vi "Check&RPN.vi"(8 "error in (no error)":errorcluster, 11 "Array STEP":T1[](array[typedef])) -> (0 "error out":errorcluster, 3 "Array STEP Out":T1[](array[typedef]))   [LabVIEW 2014, in "SeqLoop.lvlib"]
uses:
  SeqLoop.lvlib
  TypeDefs/STEP.ctl
  TypeDefs/LogicParsedExpression.ctl
  Mimico Display/TypeDefs/Mimic Data.ctl
  Mimico Display/TypeDefs/BG Image.ctl
  Mimico Display/TypeDefs/mObject.ctl
  Mimico Display/Mimico Display.lvlib
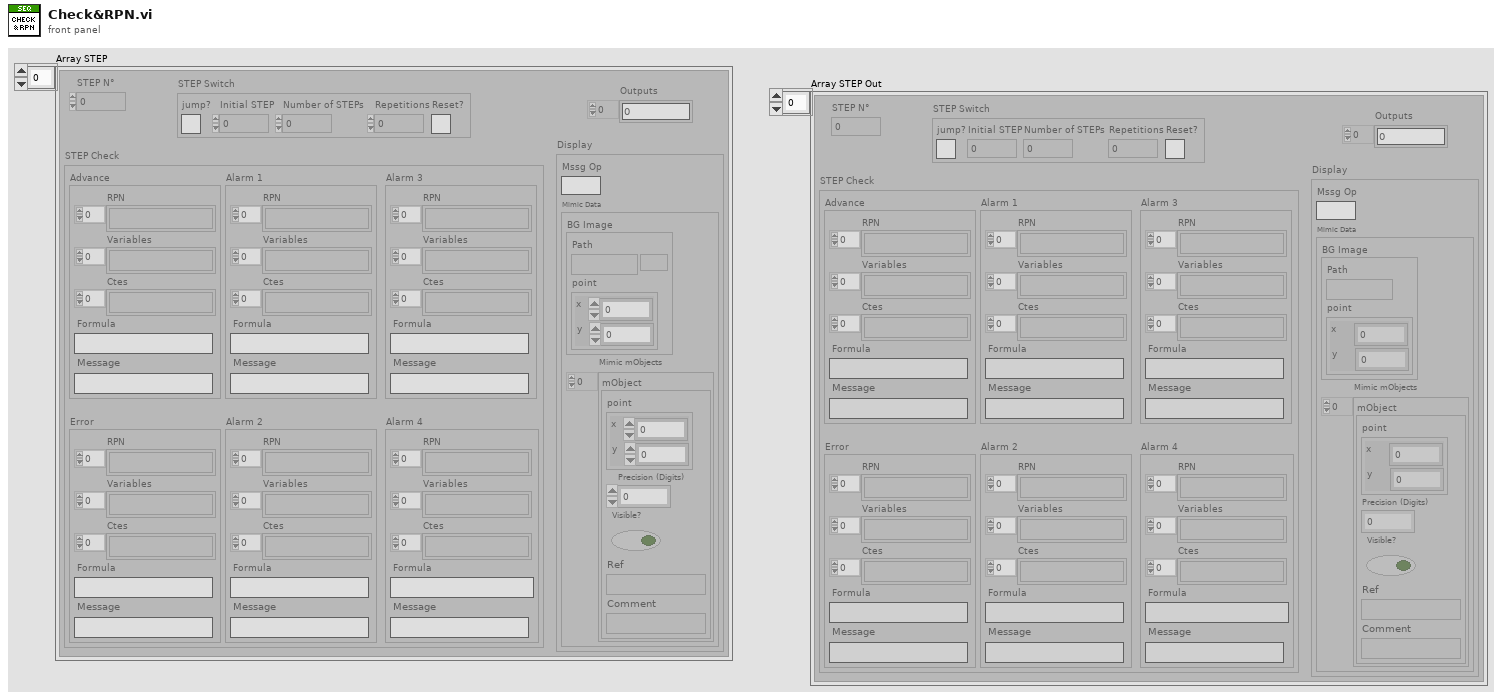
[diagram p1: front panel]
types:
  T1 = typedef "SeqLoop.lvlib/STEP.ctl" = cluster{"STEP N°":u32, "STEP Switch":cluster{"jump?":bool, "Initial STEP":u32, "Number of STEPs":u32, "Repetitions":u32, "Reset?":bool}, "Outputs":i32[], "STEP Check":cluster{"Advance":T2, "Error ":T2, "Alarm 1":T2, "Alarm 2":T2, "Alarm 3":T2, "Alarm 4":T2}, "Display":cluster{"Mssg Op":string, "Mimic Data":T3}}
  T2 = typedef "SeqLoop.lvlib/LogicParsedExpression.ctl" = cluster{"RPN ":string[], "Variables":string[], "Ctes":string[], "Formula":string, "Message":string}
  T3 = typedef "SeqLoop.lvlib/Mimico Display.lvlib/Mimic Data.ctl" = cluster{"BG Image":T4, "Mimic mObjects":T5[]}
  T4 = typedef "SeqLoop.lvlib/Mimico Display.lvlib/BG Image.ctl" = cluster{"Path":path, "point":cluster{"x":i16, "y":i16}}
  T5 = typedef "SeqLoop.lvlib/Mimico Display.lvlib/mObject.ctl" = cluster{"point":cluster{"x":i16, "y":i16}, "Precision (Digits)":i32, "Visible?":bool, "Ref":string, "Comment":string}
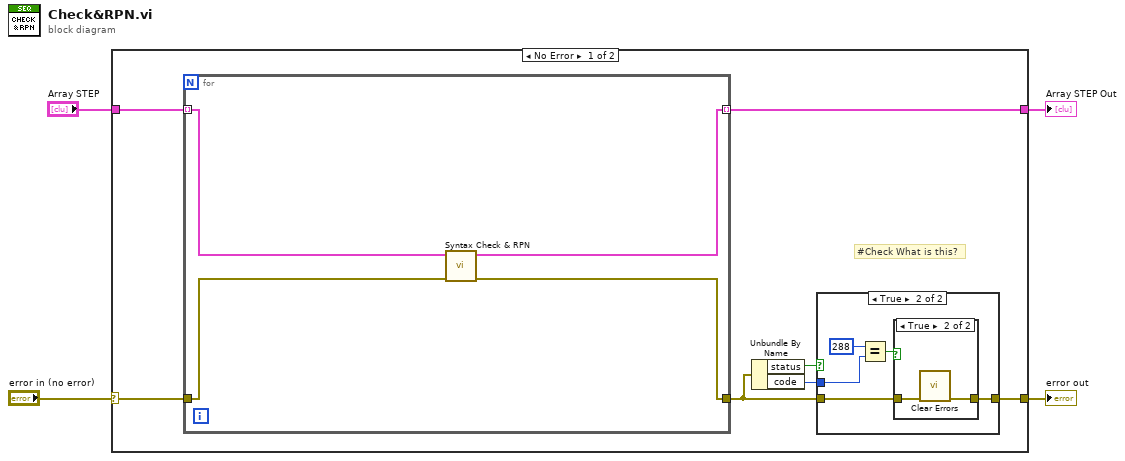
[diagram p0: block diagram]
diagram:
  n1 = case shown="No Error" "error in (no error)" {
    selector: "error in (no error)" -> [w5 w26]
    tunnel: [w8 w26] -> w3
    tunnel: "Array STEP" -> [w6 w25]
    tunnel: [w11 w25] -> w1
    frame No Error {
      # "#Check What is this?"
      n2 = for {
        tunnel: w5 -> [w24]
        tunnel: [w23] -> w7
        tunnel: w6 -> [w22] mode=indexing
        tunnel: [w21] -> w11 mode=indexing
        n3 = call "Syntax Check & RPN.vi"("error in (no error)"=w24, "STEP in"=w22) -> ("error out"=w23:errorcluster, "STEP out"=w21:T1)  [unwired: 8 in]
      }
      n4 = Unbundle By Name(w7) -> ("status"=w9:bool, "code"=w10:i32)
      n5 = case shown="True" w9 {
        tunnel: [w12 w13] -> w8
        tunnel: w7 -> [w12 w14]
        tunnel: w10 -> [_ w17]
        frame False {
        }
        frame True {
          n6 = Equal?(x=288, y=w17) -> (x = y?=w15:bool)
          n7 = case shown="True" w15 {
            tunnel: w14 -> [w18 w20]
            tunnel: [w18 w19] -> w13
            frame False {
            }
            frame True {
              n8 = call <vilib>:"Clear Errors.vi"("error in (no error)"=w20) -> ("error out"=w19:errorcluster)  [unwired: 5 in, 1 out]
            }
          }
        }
      }
    }
    frame Error {
    }
  }
  "error out" <- w3
  "Array STEP Out" <- w1
